vi "Handle Listener Result.vi"(8 "error in (no error)":errorcluster, 10 "Listener Result":T1, 11 "Websocket Server in":refnum<class "Websocket Server.lvclass">) -> (0 "error out":errorcluster, 2 "Shutdown":bool, 3 "Websocket Server out":refnum<class "Websocket Server.lvclass">)   [LabVIEW 2020, in "Stream-Websocket.lvlib" / "Websocket Server.lvclass"]
uses:
  Websocket Server.lvclass
  Websocket Server.lvclass/Websocket Server.ctl
  Listener Status.ctl
  Stream-Websocket.lvlib
  Websocket Client/Websocket Client.lvclass
  Listener Result.ctl
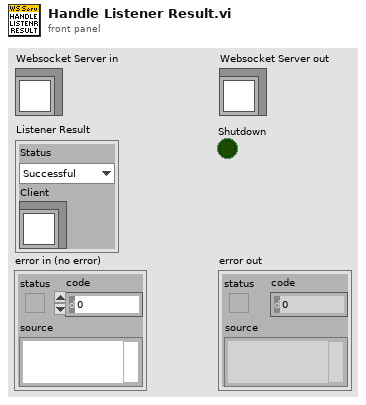
[diagram p1: front panel]
types:
  T1 = typedef "Stream-Websocket.lvlib/Listener Result.ctl" = cluster{"Status":T2, "Client":refnum<class "Websocket Client.lvclass">}
  T2 = typedef "Stream-Websocket.lvlib/Listener Status.ctl" = enum16{"Successful", "Unsuccessful"}
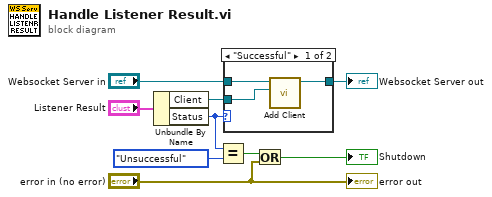
[diagram p0: block diagram]
diagram:
  n1 = Unbundle By Name("Listener Result") -> ("Client"=w3:refnum<class "Websocket Client.lvclass">, "Status"=w4:T2)
  n2 = Equal?(x=w4, y=Listener_Status."Unsuccessful") -> (x = y?=w7:bool)
  n3 = case shown="\"Successful\"" w4 {
    tunnel: w3 -> [w11 _]
    tunnel: "Websocket Server in" -> [w12 w13]
    tunnel: [w10 w13] -> w1
    frame "Successful" {
      n4 = call "Add Client.vi"("Client"=w11, "Websocket Server in"=w12) -> ("Websocket Server out"=w10:refnum<class "Websocket Server.lvclass">)  [unwired: 8 in, 1 out]
    }
    frame "Unsuccessful" {
    }
  }
  "Websocket Server out" <- w1
  n5 = Or(x=w7, y="error in (no error)") -> (x .or. y?=→"Shutdown":bool)
  "error out" <- "error in (no error)"
